vi "op_num_v6.vi"() -> ()   [LabVIEW 2009]
panel:
  out "Putere -W":dbl
  out "Kwatt-meter":dbl(knob) scale=0.0..15.0
  in  "Curent":dbl(knob) scale=0.0..50.0
  in  "Tensiune":dbl(knob) scale=0.0..250.0
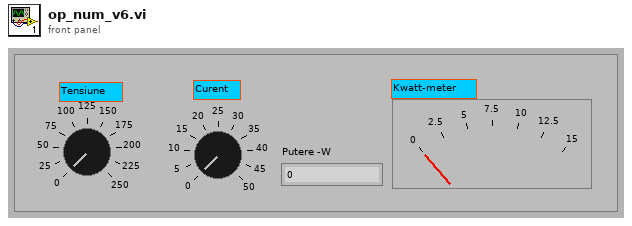
[diagram p1: front panel]
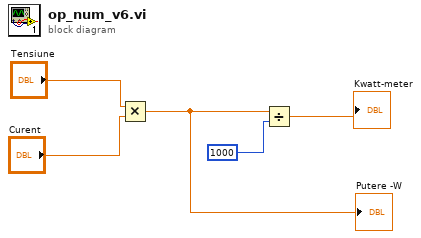
[diagram p0: block diagram]
diagram:
  n1 = Multiply(x="Tensiune", y="Curent") -> (x*y=w3:dbl)
  "Putere -W" <- w3
  n2 = Divide(x=w3, y=1000) -> (x/y=→"Kwatt-meter":dbl)
